vi "Word Search - mod.vi"(7 "Solver Selector":T1, 10 "Word List":string[](array[string])=["YELLOW", "ORANGE", "PURPLE", "BLUE", "GREEN", "RED"], 11 "Word Search Grid":string[][](array[string])=[["R", "B", "L", "U", "E", "W"], ["E", "G", "N", "A", "R", "O"], ["D", "B", "C", "E", "W", "L"], ["L", "L", "D", "K", "V", "L"], ["P", "U", "R", "P", "L", "E"], ["N", "E", "E", "R", "G", "Y"]]) -> (1 "All Words Found":bool, 2 "Execution Time":dbl)   [LabVIEW 2022 SP3]
uses:
  Solver Selector.ctl
panel:
  # "Use this Test Harness VI to time your Word Search solution (and ensure it works correctly)."
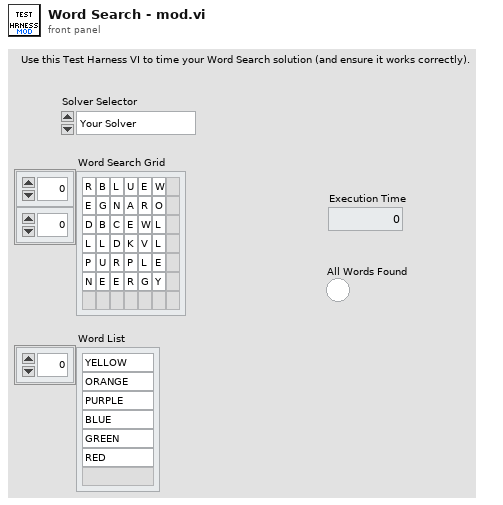
[diagram p1: front panel]
types:
  T1 = typedef "Solver Selector.ctl" = enum16{"Your Solver", "Example Solver", "Solver 001"}
  T2 = typedef "Solutions--map.ctl" = map{string, T3[]}
  T3 = typedef "Letter Index--cluster.ctl" = cluster{"Row":i32, "Column":i32}
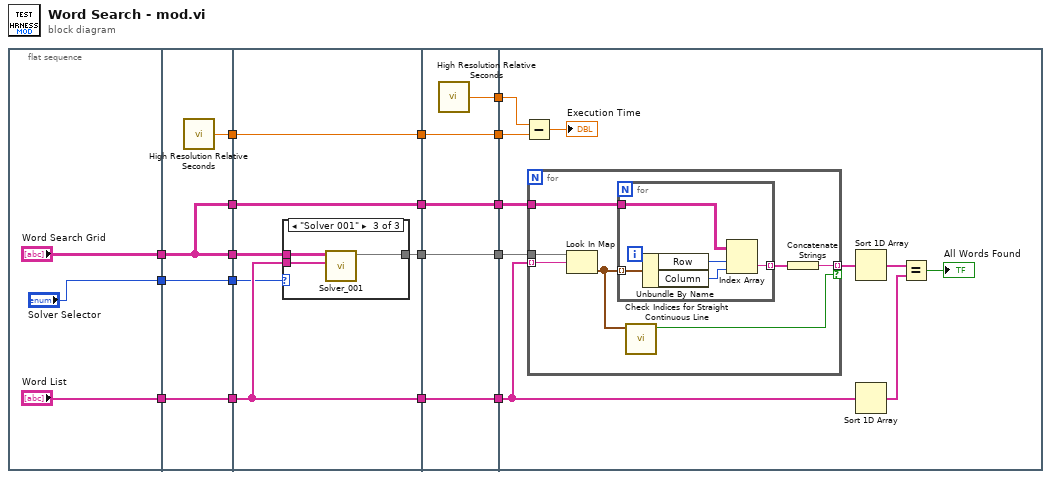
[diagram p0: block diagram]
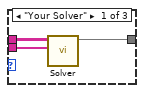
[diagram p2: hidden frame]
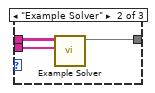
[diagram p3: hidden frame]
diagram:
  n1 = flat-sequence {
    tunnel: ["Word Search Grid"] -> w17
    tunnel: ["Word List"] -> w16
    tunnel: ["Solver Selector"] -> w1
    tunnel: w17 -> [w22]
    tunnel: w16 -> [w24]
    tunnel: [w24] -> w15
    tunnel: [w22] -> w14
    tunnel: [w23] -> w10
    tunnel: [w22] -> w3
    tunnel: [w21] -> w2
    tunnel: w1 -> [w21]
    tunnel: w15 -> [w27]
    tunnel: w14 -> [w30]
    tunnel: [w29] -> w13
    tunnel: w10 -> [w28]
    tunnel: [w28] -> w9
    tunnel: [w27] -> w6
    tunnel: [w26] -> w4
    tunnel: w3 -> [w26]
    tunnel: w2 -> [w25]
    tunnel: w13 -> [w44]
    tunnel: [w44] -> w12
    tunnel: [w43] -> w11
    tunnel: w9 -> [w42]
    tunnel: [w42] -> w8
    tunnel: [w41] -> w7
    tunnel: w6 -> [w41]
    tunnel: [w40] -> w5
    tunnel: w4 -> [w40]
    tunnel: w12 -> [w51]
    tunnel: w11 -> [w54]
    tunnel: w8 -> [w53]
    tunnel: w7 -> [w48]
    tunnel: w5 -> [w50]
    frame #0 {
    }
    frame #1 {
      n2 = call <vilib>:"High Resolution Relative Seconds.vi"() -> ("relative seconds"=w23:dbl)
    }
    frame #2 {
      n3 = case shown="\"Solver 001\"" w25 {
        tunnel: w30 -> [w33 w36 w39]
        tunnel: [w31 w35 w37] -> w29
        tunnel: w27 -> [w32 w34 w38]
        frame "Your Solver" {
          n4 = call "Solver.vi"("Word List"=w32, "Word Search Grid"=w33) -> ("Solutions"=w31:T2)  [unwired: 9 in]
        }
        frame "Example Solver" {
          n5 = call "Example Solver.vi"("Word List"=w34, "Word Search Grid"=w36) -> ("Solutions"=w35:T2)  [unwired: 9 in]
        }
        frame "Solver 001" {
          n6 = call "Solver_001.vi"("Word List"=w38, "Word Search Grid"=w39) -> ("Solutions"=w37:T2)  [unwired: 9 in]
        }
      }
    }
    frame #3 {
      n7 = call <vilib>:"High Resolution Relative Seconds.vi"() -> ("relative seconds"=w43:dbl)
    }
    frame #4 {
      n8 = Subtract(x=w54, y=w53) -> (x-y=→"Execution Time":dbl)
      n9 = for {
        tunnel: w48 -> [w60] mode=indexing
        tunnel: w51 -> [w61]
        tunnel: w50 -> [w59]
        tunnel: [w57] -> w49 mode=indexing if=w55
        n10 = Look In Map(map=w61, key=w60) -> (value=w56:T3[])  [unwired: 1 in, 1 out]
        n11 = for {
          tunnel: w56 -> [w66] mode=indexing
          tunnel: w59 -> [w64]
          tunnel: [w62] -> w58 mode=indexing
          n12 = Unbundle By Name(w66) -> ("Row"=w65:i32, "Column"=w63:i32)
          n13 = Index Array(array=w64, index (row)=w65, index (col)=w63) -> (element=w62:string)
        }
        n14 = call "Check Indices for Straight Continuous Line.vi"("Letter Indices"=w56) -> ("Straight Continuous Line?"=w55:bool)  [unwired: 10 in]
        n15 = Concatenate Strings(w58) -> (w57:string)
      }
      n16 = Sort 1D Array(array=w49) -> (sorted array=w47:string[])
      n17 = Sort 1D Array(array=w48) -> (sorted array=w46:string[])
      n18 = Equal?(x=w47, y=w46) -> (x = y?=→"All Words Found":bool)
    }
  }
